vi "test flatten tree.vi"() -> ()   [LabVIEW 2025]
uses:
  Trunk/Configuration Framework/serializable configuration/NISE_CEF_serializable configuration.lvclass
  Trunk/Configuration Framework/tree serializer/hierarchy element.ctl
  Trunk/Configuration Framework/tree serializer/memory hierarchy.ctl
  Trunk/Configuration Framework/tree serializer/full hierarchy.ctl
panel:
  out "memory hierarchy out":T1
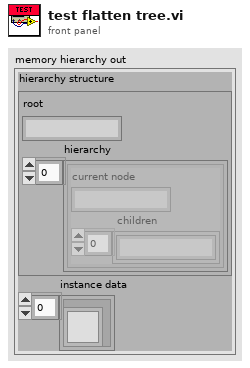
[diagram p1: front panel]
types:
  T1 = typedef "NISE_CEF_TreeSerializer.lvlib/memory hierarchy.ctl" = cluster{"hierarchy structure":T2, "instance data":refnum<class "NISE_CEF_serializable configuration.lvclass">[]}
  T2 = typedef "NISE_CEF_TreeSerializer.lvlib/full hierarchy.ctl" = cluster{"root":string, "hierarchy":T3[]}
  T3 = typedef "NISE_CEF_TreeSerializer.lvlib/hierarchy element.ctl" = cluster{"current node":string, "children":string[]}
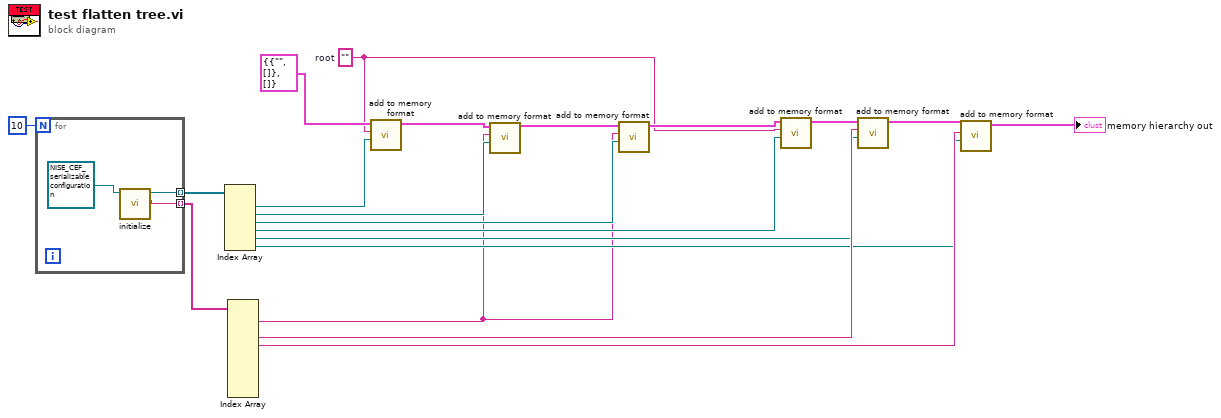
[diagram p0: block diagram]
diagram:
  w10 = ""  # root
  n1 = for {
    N: 10 -> [_]
    tunnel: [w22] -> w17 mode=indexing
    tunnel: [w21] -> w18 mode=indexing
    n2 = call "initialize.vi"("configuration in"=refnum<class "NISE_CEF_serializable configuration.lvclass"> refnum ("configuration")) -> ("identifier"=w22:string, "configuration out"=w21:refnum<class "NISE_CEF_serializable configuration.lvclass">)  [unwired: 8 in, 1 out]
  }
  n3 = Index Array(array=w18) -> (element #1=w14:refnum<class "NISE_CEF_serializable configuration.lvclass">, element #2=w12:refnum<class "NISE_CEF_serializable configuration.lvclass">, element #3=w13:refnum<class "NISE_CEF_serializable configuration.lvclass">, element #4=w9:refnum<class "NISE_CEF_serializable configuration.lvclass">, element #5=w4:refnum<class "NISE_CEF_serializable configuration.lvclass">, element #6=w2:refnum<class "NISE_CEF_serializable configuration.lvclass">)  [unwired: 6 in]
  n4 = Index Array(array=w17) -> (element #1=w1:string, element #3=w5:string, element #4=w3:string)  [unwired: 10 in, 7 out]
  n5 = call "add to memory format.vi"("NISE_CEF_serializable configuration in"=w14, "parent ID"=w10, "memory hierarchy in"=T1 {"hierarchy structure"={"root"="", "hierarchy"=[]}, "instance data"=[]} ("memory hierarchy out")) -> ("memory hierarchy out"=w15:T1)  [unwired: 7 in, 1 out]
  n6 = call "add to memory format.vi"("NISE_CEF_serializable configuration in"=w12, "parent ID"=w1, "memory hierarchy in"=w15) -> ("memory hierarchy out"=w16:T1)  [unwired: 7 in, 1 out]
  n7 = call "add to memory format.vi"("NISE_CEF_serializable configuration in"=w13, "parent ID"=w1, "memory hierarchy in"=w16) -> ("memory hierarchy out"=w11:T1)  [unwired: 7 in, 1 out]
  n8 = call "add to memory format.vi"("NISE_CEF_serializable configuration in"=w9, "parent ID"=w10, "memory hierarchy in"=w11) -> ("memory hierarchy out"=w8:T1)  [unwired: 7 in, 1 out]
  n9 = call "add to memory format.vi"("NISE_CEF_serializable configuration in"=w4, "parent ID"=w5, "memory hierarchy in"=w8) -> ("memory hierarchy out"=w7:T1)  [unwired: 7 in, 1 out]
  n10 = call "add to memory format.vi"("NISE_CEF_serializable configuration in"=w2, "parent ID"=w3, "memory hierarchy in"=w7) -> ("memory hierarchy out"=→"memory hierarchy out":T1)  [unwired: 7 in, 1 out]
